vi "Set Level.vi"(6 "Output Channel":T1, 8 "error in (no error)":errorcluster, 9 "Slew (V/s)":dbl, 10 "Level (V)":dbl, 11 "Inst.RP100 in":refnum<class "Inst.RP100.lvclass">) -> (0 "error out":errorcluster, 3 "Inst.RP100 out":refnum<class "Inst.RP100.lvclass">)   [LabVIEW 2019, in "Inst.RP100.lvlib" / "Inst.RP100.lvclass"]
doc: "Set the output <b>Level</b> with <b>Slew</b> rate on the selected <b>Output Channel</b>"
uses:
  Inst.RP100.lvclass
  Typedefs/Channel--Num.ctl
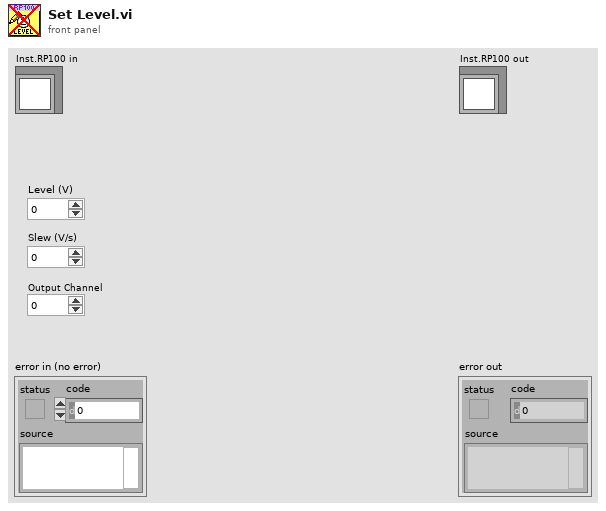
[diagram p1: front panel]
types:
  T1 = typedef "Inst.RP100.lvlib/Inst.RP100.lvclass/Channel--Num.ctl" = i32
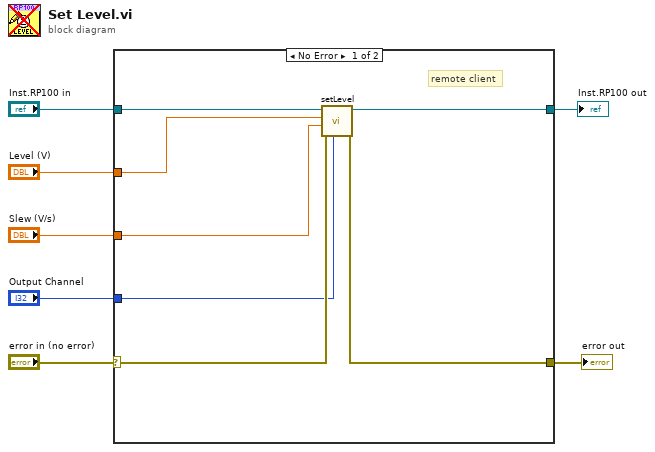
[diagram p0: block diagram]
diagram:
  n1 = case shown="No Error" "error in (no error)" {
    selector: "error in (no error)" -> [w11 w16]
    tunnel: [w9 w16] -> w6
    tunnel: "Level (V)" -> [w10 _]
    tunnel: "Inst.RP100 in" -> [w13 w15]
    tunnel: [w12 w15] -> w3
    tunnel: "Slew (V/s)" -> [w14 _]
    tunnel: "Output Channel" -> [w8 _]
    frame No Error {
      # "remote client"
      n2 = call-dynamic "setLevel.vi"("Output Channel"=w8, "error in (no error)"=w11, "Slew (V/s)"=w14, "Level (V)"=w10, "Inst.RP100 in"=w13) -> ("error out"=w9:errorcluster, "Inst.RP100 out"=w12:refnum<class "Inst.RP100.lvclass">)  [unwired: 5 in]
    }
    frame Error {
    }
  }
  "error out" <- w6
  "Inst.RP100 out" <- w3
